vi "Is there an Error.vi"(2 "Error In":errorcluster) -> (7 "Error?":bool)   [LabVIEW 2021, in "Error.lvlib"]
uses:
  Error.lvlib
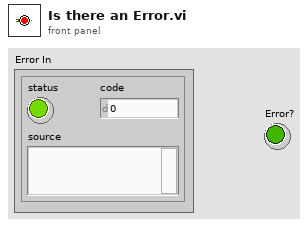
[diagram p1: front panel]
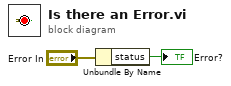
[diagram p0: block diagram]
diagram:
  n1 = Unbundle By Name("Error In") -> ("status"=→"Error?":bool)
